vi "CmdConsole.Init.vi"(6 "WorkingDir":path, 8 "error in (no error)":errorcluster, 9 "Args":string, 10 "App":path, 11 "CmdConsole in":refnum<class "CmdConsole.lvclass">) -> (0 "error out":errorcluster, 3 "CmdConsole out":refnum<class "CmdConsole.lvclass">)   [LabVIEW 2024, in "CmdConsole.lvclass"]
uses:
  CmdConsole.lvclass
  CmdConsole.lvclass/CmdConsole.ctl
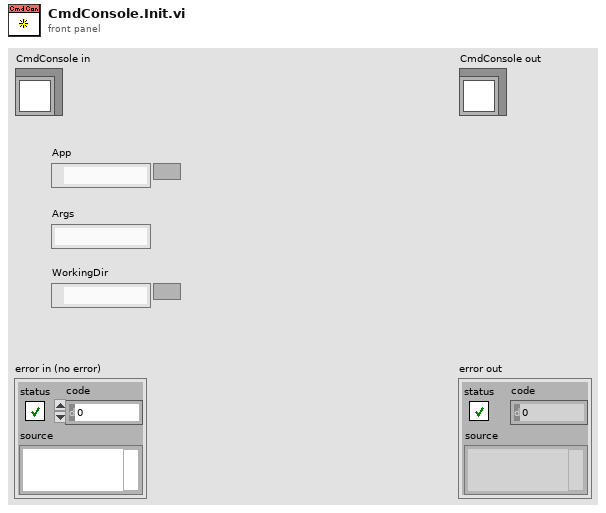
[diagram p1: front panel]
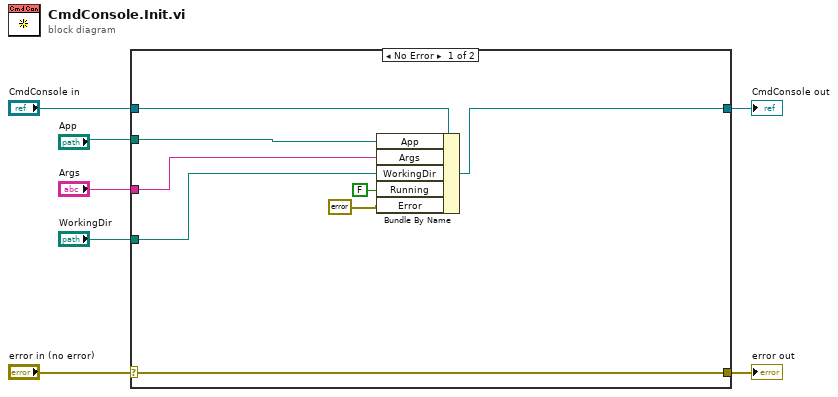
[diagram p0: block diagram]
diagram:
  n1 = case shown="No Error" "error in (no error)" {
    selector: "error in (no error)" -> [w15 w17]
    tunnel: [w15 w17] -> w6
    tunnel: [w13 w16] -> w4
    tunnel: "CmdConsole in" -> [w14 w16]
    tunnel: "App" -> [w12 _]
    tunnel: "Args" -> [w11 _]
    tunnel: "WorkingDir" -> [w10 _]
    frame No Error {
      n2 = Bundle By Name(cluster=w14, "App"=w12, "Args"=w11, "WorkingDir"=w10, "Running"=FALSE, "Error"=errorcluster {"status"=FALSE, "code"=0, "source"=""}) -> (w13:refnum<class "CmdConsole.lvclass">)
    }
    frame Error {
    }
  }
  "error out" <- w6
  "CmdConsole out" <- w4
